vi "FM-Bessel.vi"() -> ()   [LabVIEW 2013]
panel:
  in  "Kf":dbl(slide) caption="Constante de proporcionalidade (Kf)" min=0.0 max=10000.0 step=100.0 scale=0.0..10000.0
  out "mod":cluster{dbl[], dbl[]}(graph) caption="Modulação"
  out "Portadora":cluster{dbl[], dbl[]}(graph)
  out "Informação":cluster{dbl[], dbl[]}(graph)
  in  "dt":dbl caption="Precisao temporal"
  in  "fm":dbl caption="Frequencia do sinal modulador"
  in  "fp":dbl caption="Frequencia da portadora"
  in  "E0":dbl caption="Amplitude da portadora"
  in  "Em":dbl caption="Amplitude do sinal modulador"
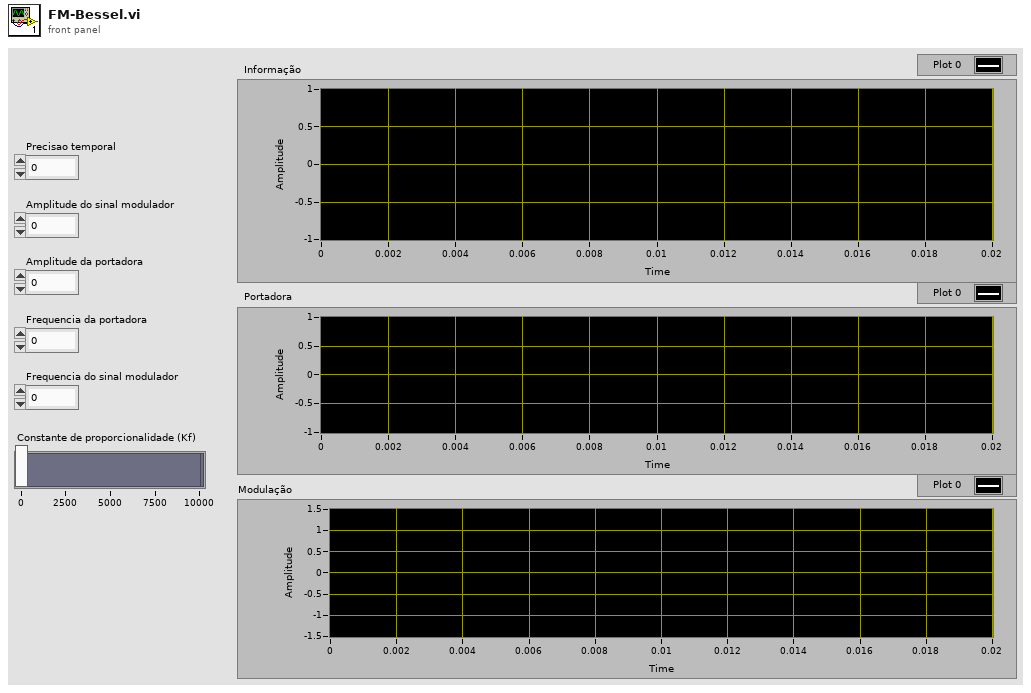
[diagram p1: front panel]
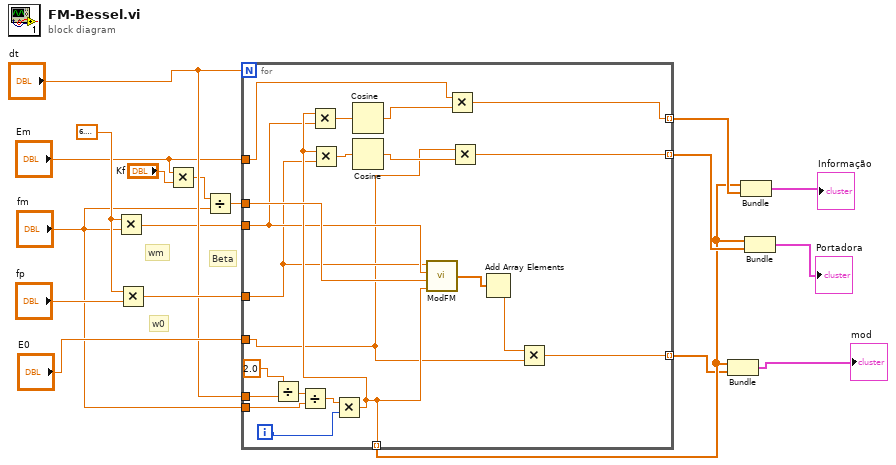
[diagram p0: block diagram]
diagram:
  w18 = 6.283185307179586
  # "wm"
  # "w0"
  # "Beta"
  n1 = Multiply(x=w18, y="fm") -> (x*y=w5:dbl)
  n2 = Multiply(x=w18, y="fp") -> (x*y=w17:dbl)
  n3 = Multiply(x="Em", y="Kf") -> (x*y=w6:dbl)
  n4 = Divide(x=w6, y="fm") -> (x/y=w4:dbl)
  n5 = for {
    N: "dt" -> [_]
    tunnel: "Em" -> [w29]
    tunnel: "E0" -> [w20]
    tunnel: w5 -> [w24]
    tunnel: w17 -> [w23]
    tunnel: "dt" -> [w39]
    tunnel: [w28] -> w14 mode=indexing
    tunnel: [w27] -> w13 mode=indexing
    tunnel: "fm" -> [w32]
    tunnel: [w25] -> w9 mode=indexing
    tunnel: w4 -> [w26]
    tunnel: [w19] -> w2 mode=indexing
    i -> [w35]
    n6 = Divide(x=2.0, y=w39) -> (x/y=w37:dbl)
    n7 = Divide(x=w37, y=w32) -> (x/y=w36:dbl)
    n8 = Multiply(x=w36, y=w35) -> (x*y=w25:dbl)
    n9 = Multiply(x=w25, y=w24) -> (x*y=w34:dbl)
    n10 = Multiply(x=w25, y=w23) -> (x*y=w33:dbl)
    n11 = Cosine(x=w34) -> (cos(x)=w31:dbl)
    n12 = Cosine(x=w33) -> (cos(x)=w30:dbl)
    n13 = call "ModFM.vi"("t"=w25, "n"=w26, "wm"=w24, "w0"=w23) -> ("et"=w22:dbl[])
    n14 = Multiply(x=w29, y=w31) -> (x*y=w28:dbl)
    n15 = Multiply(x=w20, y=w30) -> (x*y=w27:dbl)
    n16 = Add Array Elements(numeric array=w22) -> (sum=w21:dbl)
    n17 = Multiply(x=w21, y=w20) -> (x*y=w19:dbl)
  }
  n18 = Bundle(w9, w2) -> (→"mod":cluster{dbl[], dbl[]})  [unwired: 1 in]
  n19 = Bundle(w9, w14) -> (→"Informação":cluster{dbl[], dbl[]})  [unwired: 1 in]
  n20 = Bundle(w9, w13) -> (→"Portadora":cluster{dbl[], dbl[]})  [unwired: 1 in]
